vi "Error Query1.vi"(8 "error in (no error)":errorcluster, 11 "VISA resource name":refnum<visa-resource-name>) -> (0 "error out":errorcluster, 1 "Error Message":string, 2 "Error Code":i32[](array[numeric]), 3 "VISA resource name out":refnum<visa-resource-name>)   [LabVIEW 2015, in "Agilent 3446X Series1.lvlib"]
doc: "Queries the instrument for any errors in the instrument's error queue. It will continue to read errors until all errors have been read from the instrument. Any errors will be returned in the <B>error out</B> control.\n\n<B>Note:</B>\nThis VI is called automatically by most driver VIs so it is not usually necessary to call this in an application."
uses:
  Agilent 3446X Series1.lvlib
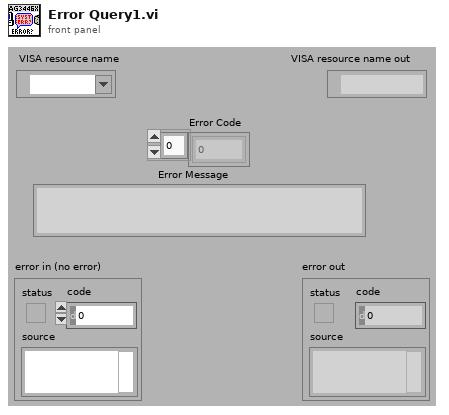
[diagram p1: front panel]
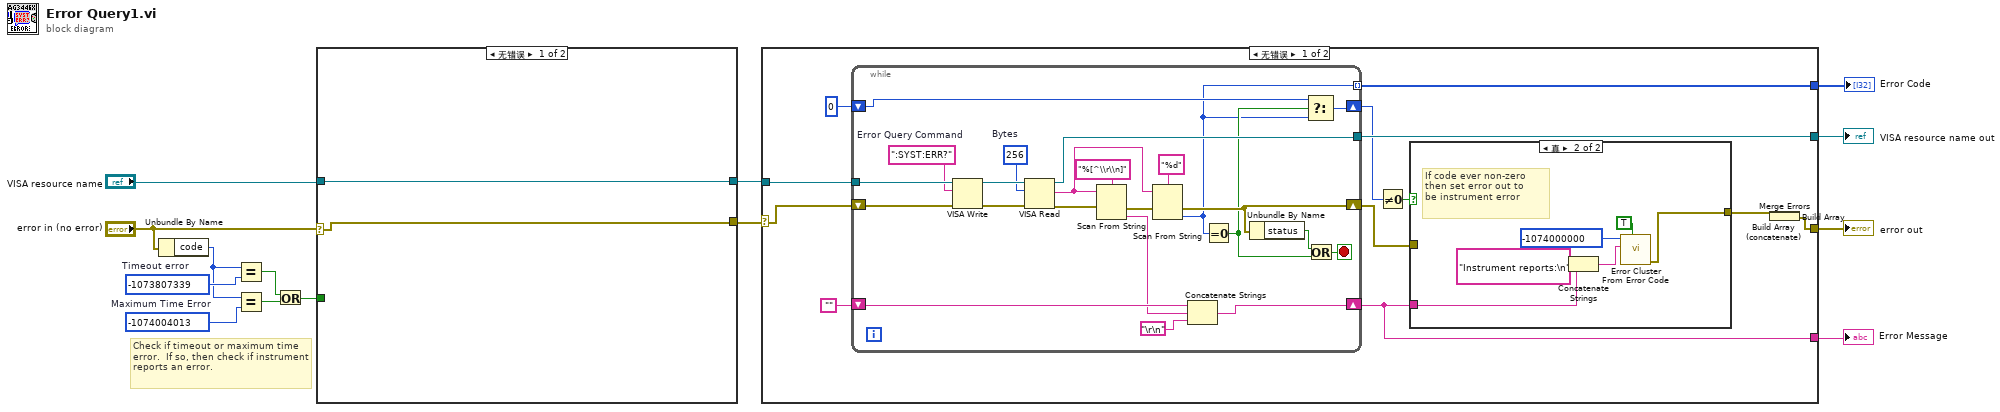
[diagram p0: block diagram]
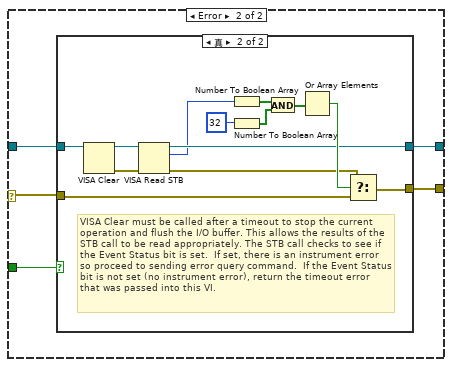
[diagram p2: hidden frame]
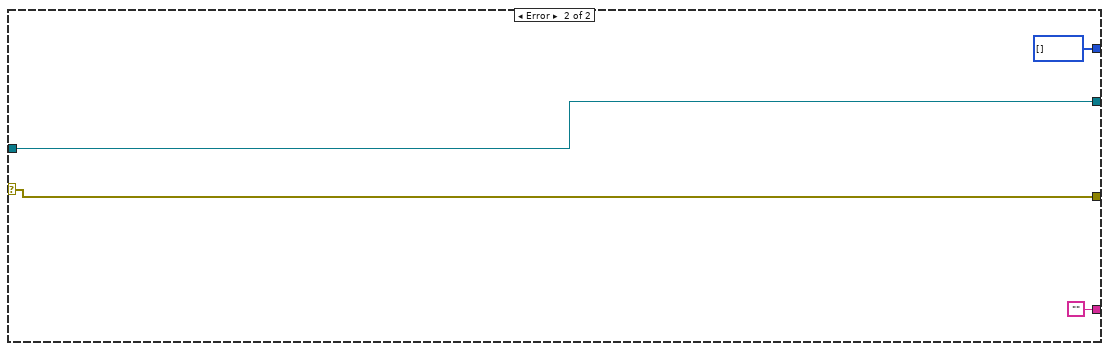
[diagram p5: hidden frame]
diagram:
  w5 = -1074004013  # Maximum Time Error
  w7 = -1073807339  # Timeout error
  # "Check if timeout or maximum time error.  If so, then check if instrument reports an error."
  n1 = Unbundle By Name("error in (no error)") -> ("code"=w6:i32)
  n2 = Equal?(x=w6, y=w7) -> (x = y?=w3:bool)
  n3 = Equal?(x=w6, y=w5) -> (x = y?=w4:bool)
  n4 = Or(x=w3, y=w4) -> (x .or. y?=w2:bool)
  n5 = case shown="无错误" "error in (no error)" {
    selector: "error in (no error)" -> [w15 w19]
    tunnel: "VISA resource name" -> [w16 w21]
    tunnel: [w16 w20] -> w9
    tunnel: [w15 w18] -> w10
    tunnel: w2 -> [_ w17]
    frame No Error {
    }
    frame Error {
      n6 = case shown="真" w17 {
        tunnel: w21 -> [w23 w29]
        tunnel: [w23 w26] -> w20
        tunnel: w19 -> [w22 w32]
        tunnel: [w22 w31] -> w18
        frame False {
          # "Error code not a timeout, so best to pass on to user."
        }
        frame True {
          # "VISA Clear must be called after a timeout to stop the current operation and flush the I/O buffer. This allows the results of the  STB call to be read appropriately. The STB call checks to see if the Event Status bit is set.  If set, there is an instrument error so proceed to sending error query command.  If the Event Status bit is not set (no instrument error), return the timeout error that was passed into this VI."
          n7 = VISA Clear(VISA resource name=w29) -> (VISA resource name out=w28:refnum<visa-resource-name>, error out=w27:errorcluster)  [unwired: 1 in]
          n8 = VISA Read STB(8:w27, 11:w28) -> (0:w25:errorcluster, 2:w24:u16, 3:w26:refnum<visa-resource-name>)
          n9 = Number To Boolean Array(number=w24) -> (Boolean array=w33:bool[])
          n10 = Number To Boolean Array(number=32) -> (Boolean array=w35:bool[])
          n11 = And(x=w33, y=w35) -> (x .and. y?=w34:bool[])
          n12 = Or Array Elements(Boolean array=w34) -> (logical OR=w30:bool)
          n13 = Select(t=w25, s=w30, f=w32) -> (s? t:f=w31:errorcluster)
        }
      }
    }
  }
  n14 = case shown="无错误" w10 {
    selector: w10 -> [w39 w81]
    tunnel: [w50 w84] -> w14
    tunnel: w9 -> [w49 w84]
    tunnel: [w47 w81] -> w13
    tunnel: [w42 ""] -> w12
    tunnel: [w41 i32[] []] -> w11
    frame No Error {
      n15 = while {
        tunnel: [w80] -> w50
        tunnel: w49 -> [w79]
        shift-right: [w67] -> w42
        shift-left: "" -> [w70]
        shift-right: [w65] -> w43
        shift-left: 0 -> [w66]
        shift-right: [w63] -> w40
        shift-left: w39 -> [w64]
        tunnel: [w58] -> w41 mode=indexing
        stop <- w73 stop-if-true
        w77 = u32 256  # Bytes
        w75 = ":SYST:ERR?"  # Error Query Command
        n16 = VISA Write(VISA resource name=w79, write buffer=w75, error in (no error)=w64) -> (VISA resource name out=w78:refnum<visa-resource-name>, error out=w76:errorcluster)  [unwired: 1 out]
        n17 = VISA Read(VISA resource name=w78, byte count=w77, error in (no error)=w76) -> (VISA resource name out=w80:refnum<visa-resource-name>, read buffer=w71:string, error out=w62:errorcluster)  [unwired: 1 out]
        n18 = Scan From String(format string="%[^\\r\\n]", input string=w71, error in=w62) -> (error out=w61:errorcluster, output 1=w68:string)  [unwired: 1 in, 3 out]
        n19 = Scan From String(format string="%d", input string=w71, error in=w61) -> (error out=w63:errorcluster, output 1=w58:i32)  [unwired: 1 in, 3 out]
        n20 = Concatenate Strings(w70, w68, "\r\n") -> (w67:string)
        n21 = Equal To 0?(x=w58) -> (x = 0?=w59:bool)
        n22 = Unbundle By Name(w63) -> ("status"=w60:bool)
        n23 = Select(t=w66, s=w59, f=w58) -> (s? t:f=w65:i32)
        n24 = Or(x=w60, y=w59) -> (x .or. y?=w73:bool)
      }
      n25 = Not Equal To 0?(x=w43) -> (x != 0?=w45:bool)
      n26 = case shown="真" w45 {
        tunnel: w42 -> [_ w56]
        tunnel: [w51 w52] -> w44
        tunnel: w40 -> [w51 _]
        frame False {
        }
        frame True {
          # "If code ever non-zero\nthen set error out to\nbe instrument error"
          n27 = Concatenate Strings("Instrument reports:\n" ("Source"), w56) -> (w53:string)
          n28 = call <vilib>:"Error Cluster From Error Code.vi"("show call chain? (False)"=TRUE, "error message (\"\")"=w53, "error code (0)"=-1074000000 ("Code")) -> ("error out"=w52:errorcluster)  [unwired: 1 in, 5 out]
        }
      }
      n29 = Build Array(w44) -> (w38:errorcluster[])
      n30 = Build Array (concatenate)(w38) -> (w37:errorcluster[])
      n31 = Merge Errors(w37) -> (w47:errorcluster)
    }
    frame Error {
    }
  }
  "VISA resource name out" <- w14
  "error out" <- w13
  "Error Message" <- w12
  "Error Code" <- w11
